vi "Write Value 2.vi"(8 "error in (no error)":errorcluster, 10 "Value":dbl, 11 "TCPController in":refnum<class "TCPController.lvclass">) -> (0 "error out":errorcluster, 3 "TCPController out":refnum<class "TCPController.lvclass">)   [LabVIEW 2020, in "TCPController.lvclass"]
uses:
  TCPController.lvclass
  TCPController.lvclass/TCPController.ctl
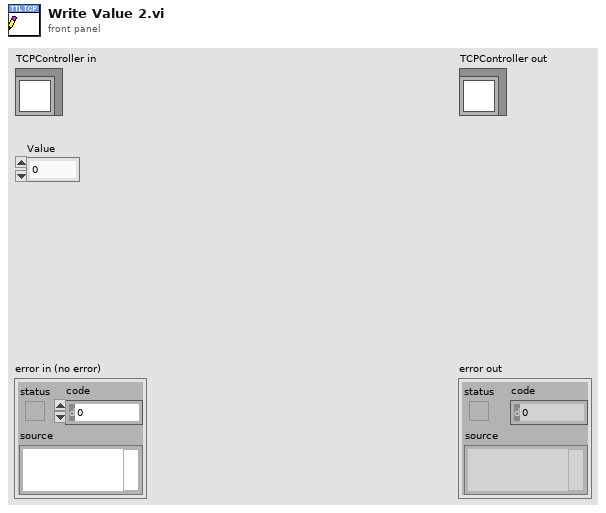
[diagram p1: front panel]
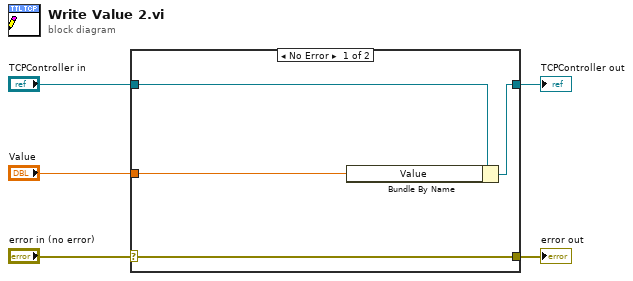
[diagram p0: block diagram]
diagram:
  n1 = case shown="No Error" "error in (no error)" {
    selector: "error in (no error)" -> [w9 w10]
    tunnel: [w9 w10] -> w4
    tunnel: [w7 w11] -> w2
    tunnel: "TCPController in" -> [w8 w11]
    tunnel: "Value" -> [w6 _]
    frame No Error {
      n2 = Bundle By Name(cluster=w8, "Value"=w6) -> (w7:refnum<class "TCPController.lvclass">)
    }
    frame Error {
    }
  }
  "error out" <- w4
  "TCPController out" <- w2
